vi "Read.vi"(8 "error in":errorcluster, 11 "Reply Protocol DataSocket in":refnum<class "Reply Protocol DataSocket.lvclass">) -> (0 "error out":errorcluster, 2 "Reply":variant, 3 "Reply Protocol DataSocket out":refnum<class "Reply Protocol DataSocket.lvclass">)   [LabVIEW 2023, in "HAL GOOP4.lvlib" / "Reply Protocol DataSocket.lvclass"]
uses:
  Reply Protocol DataSocket.lvclass
  Reply Protocol Base/Reply Protocol Base.lvclass/Reply Protocol Base.ctl
  Reply Protocol DataSocket.lvclass/Reply Protocol DataSocket.ctl
  Reply Protocol Base/Reply Protocol Base.lvclass
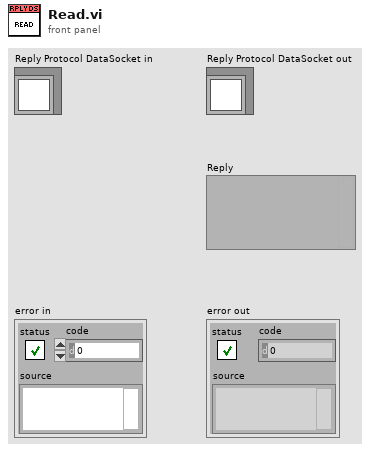
[diagram p1: front panel]
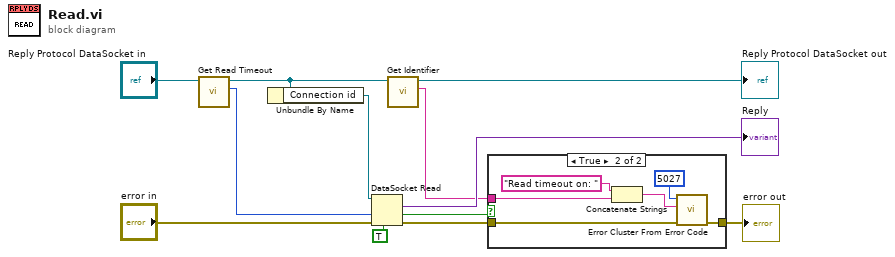
[diagram p0: block diagram]
diagram:
  n1 = call "Get Read Timeout.vi"("Reply Protocol Base in"="Reply Protocol DataSocket in") -> ("Read Timeout"=w3:i32, "Reply Protocol Base out"=w4:refnum<class "Reply Protocol DataSocket.lvclass">)  [unwired: 9 in]
  n2 = Unbundle By Name(w4) -> ("Connection id"=w5:refnum<k13>)
  n3 = DataSocket Read(6:TRUE ("wait for updated value (T)"), 8:"error in", 9:w3, 11:w5) -> (0:w8:errorcluster, 1:w9:bool, 2:→"Reply":variant)  [unwired: 1 in, 4 out]
  n4 = call "Get Identifier.vi"("Reply Protocol Base in"=w4) -> ("Identifier"=w1:string, "Reply Protocol Base out"=→"Reply Protocol DataSocket out":refnum<class "Reply Protocol DataSocket.lvclass">)  [unwired: 9 in]
  n5 = case shown="True" w9 {
    tunnel: w8 -> [w13 w18]
    tunnel: [w13 w19] -> w7
    tunnel: w1 -> [_ w14]
    frame False {
    }
    frame True {
      n6 = Concatenate Strings("Read timeout on: " ("string"), w14) -> (w16:string)
      n7 = call <vilib>:"Error Cluster From Error Code.vi"("error in (no error)"=w18, "error message (\"\")"=w16, "error code (0)"=5027) -> ("error out"=w19:errorcluster)  [unwired: 6 in]
    }
  }
  "error out" <- w7
